vi "RT Error Handler - Acquisition and Logging.vi"(7 "Stop FPGA Timeout":bool, 8 "error in (no error)":errorcluster, 10 "IRQ Timeout":bool, 11 "Message Queue":refnum<queue>) -> (3 "dup Message Queue":refnum<queue>)   [LabVIEW 2020]
uses:
  support/Message Queue/Message Cluster.ctl
  support/Message Queue/Message Queue.lvlib
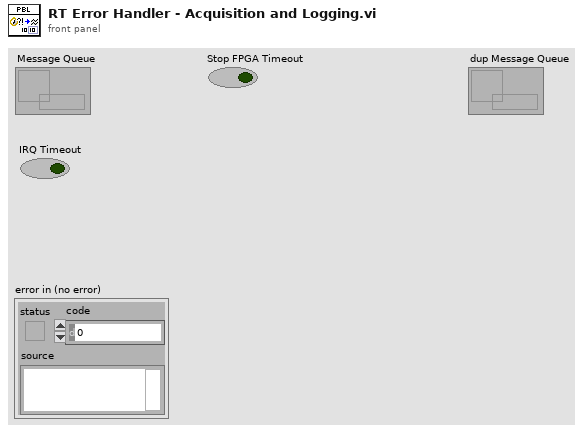
[diagram p1: front panel]
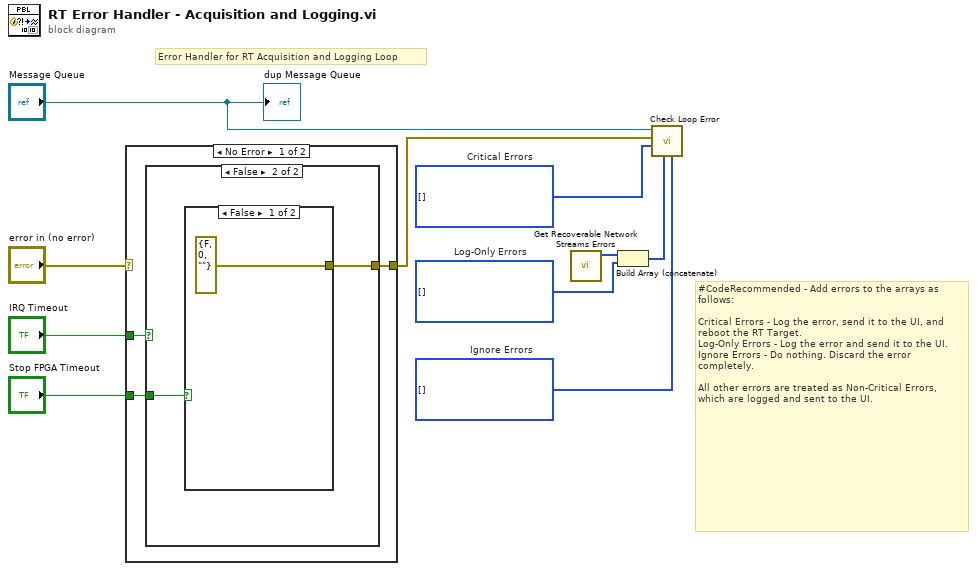
[diagram p0: block diagram]
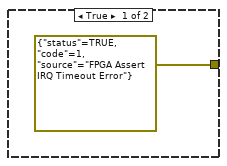
[diagram p2: hidden frame]
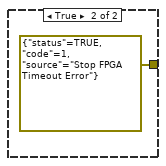
[diagram p3: hidden frame]
diagram:
  w9 = i32[] []  # Ignore Errors
  w3 = i32[] []  # Log-Only Errors
  w10 = i32[] []  # Critical Errors
  # "#CodeRecommended - Add errors to the arrays as follows:\n\nCritical Errors - Log the error, send it to the UI, and reboot the RT Target.\nLog-Only Errors - Log the error and send it to the UI.\nIgnore Errors - Do nothing. Discard the error completely.\n\nAll other errors are treated as Non-Critical Errors, which are logged and sent to the UI."
  # "Error Handler for RT Acquisition and Logging Loop"
  n1 = case shown="No Error" "error in (no error)" {
    selector: "error in (no error)" -> [_ w19]
    tunnel: "IRQ Timeout" -> [w13 _]
    tunnel: [w12 w19] -> w5
    tunnel: "Stop FPGA Timeout" -> [w11 _]
    frame No Error {
      n2 = case shown="False" w13 {
        tunnel: [errorcluster {"status"=TRUE, "code"=1, "source"="FPGA Assert IRQ Timeout Error"} ("error constant") w16] -> w12
        tunnel: w11 -> [_ w15]
        frame True {
        }
        frame False {
          n3 = case shown="False" w15 {
            tunnel: [errorcluster {"status"=FALSE, "code"=0, "source"=""} ("error constant") errorcluster {"status"=TRUE, "code"=1, "source"="Stop FPGA Timeout Error"} ("error constant")] -> w16
            frame False {
            }
            frame True {
            }
          }
        }
      }
    }
    frame Error {
    }
  }
  n4 = call "Get Recoverable Network Streams Errors.vi"() -> ("recoverable network streams errors"=w4:i32[])  [unwired: 11 in]
  n5 = Build Array (concatenate)(w4, w3) -> (w2:i32[])
  n6 = call "Check Loop Error.vi"("Ignore Errors"=w9, "Log-Only Errors"=w2, "Critical Errors"=w10, "error to process"=w5, "Message Queue"="Message Queue") -> ()  [unwired: 5 in, 2 out]
  "dup Message Queue" <- "Message Queue"
